vi "SimpleSetMotor.vi"(8 "error in (no error)":errorcluster, 10 "Output":dbl, 11 "MotorControlDevRef":T1={"DeviceStatus"={"status"=FALSE, "code"=0, "source"=""}, "Type"=enum."PWM", "PWM"={"Digital Module"=enum."Digital Module 1", "PWM Channel"=enum."Invalid", "DeadBand"={"Name"="", "maxPositivePwm"=0, "minPositivePwm"=0, "centerPwm"=0, "maxNegativePwm"=0, "minNegativePwm"=0, "angularRange"=0}}, "CAN"={"Device Number"=0, "Control Mode"=enum."Percent VBus", "Semaphore"=refnum, "Max Vout"=12.0}, "Invert"=FALSE, "TransformRef"=refnum, "InvTransformRef"=refnum}) -> (0 "error out":errorcluster, 3 "MotorControlDevRef":T1={"DeviceStatus"={"status"=FALSE, "code"=0, "source"=""}, "Type"=enum."PWM", "PWM"={"Digital Module"=enum."Digital Module 1", "PWM Channel"=enum."Invalid", "DeadBand"={"Name"="", "maxPositivePwm"=0, "minPositivePwm"=0, "centerPwm"=0, "maxNegativePwm"=0, "minNegativePwm"=0, "angularRange"=0}}, "CAN"={"Device Number"=0, "Control Mode"=enum."Percent VBus", "Semaphore"=refnum, "Max Vout"=12.0}, "Invert"=FALSE, "TransformRef"=refnum, "InvTransformRef"=refnum})   [LabVIEW 2011]
doc: "Specifies the output value or set-point for the motor controller.\n\nIf you use a Jaguar or Victor motor controller connected to PWM, the scaled value can range from -1.0 to 1.0.\n\nIf you use a CAN Jaguar, the scale and the units depend on the mode the Jaguar is in. In <B>Percent VBus</B> mode, the range is the same as the PWM interface. In <B>Voltage</B>, <B>Current</B>, <B>Speed</B>, and <B>Position</B> modes, the <B>Output</B> is specified in engineering units (Volts, Amps, Rotations/Minute, and Rotations respectively).\n\nThe output value can be modified by custom scaling if you specify the <B>TransformRef</B> VI reference in the Open VI. Use this transform if you need to apply a non-linear transformation to the motor control signal to compensate for the characteristics of the motor.\n\nThis software is licensed. Open the labview\\readme\\WPI Robotics Library Open Source License.txt file for more information."
uses:
  <vilib>/Rock Robotics/WPI/MotorControl/WPI_MotorControlDeviceRef.ctl
  <vilib>/Rock Robotics/SystemInterfaces/Typedef/FPGA_TypedefDigitalModule.ctl
  <vilib>/Rock Robotics/SystemInterfaces/DIO/FPGA_DIOPWMChannel.ctl
  <vilib>/Rock Robotics/WPI/PWM/WPI_PWMDeadband.ctl
  <vilib>/Rock Robotics/WPI/CAN/Jaguar/SubVIs/WPI_CANJaguar_ControlMode.ctl
  <vilib>/Rock Robotics/WPI/PWM/WPI_PWMTransform_ConPane.ctl
  <vilib>/Rock Robotics/SystemInterfaces/DIO/FPGA_DIODevRef.ctl
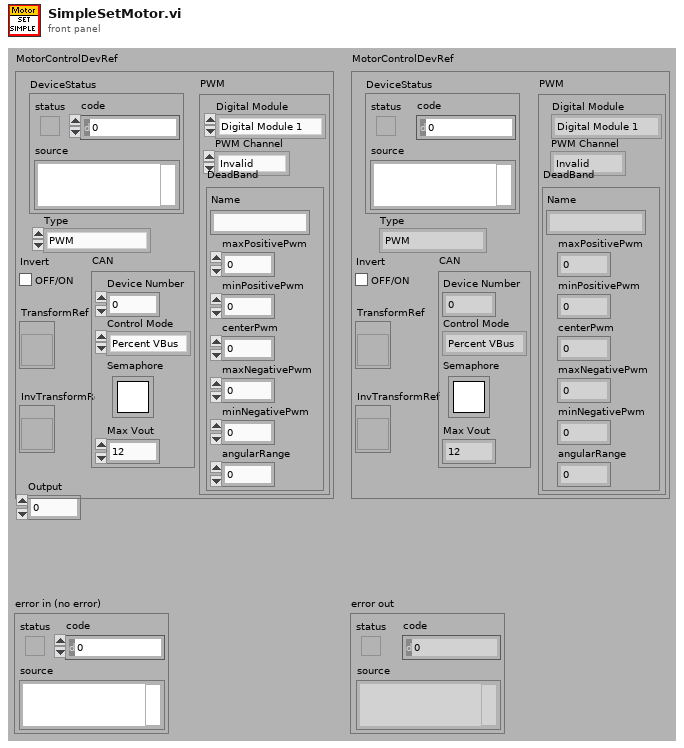
[diagram p1: front panel]
types:
  T1 = typedef "WPI_MotorControlDeviceRef.ctl" = cluster{"DeviceStatus":errorcluster, "Type":enum16{"PWM", "CAN"}, "PWM":cluster{"Digital Module":T2, "PWM Channel":T3, "DeadBand":T4}, "CAN":cluster{"Device Number":u8, "Control Mode":T5, "Semaphore":T6, "Max Vout":dbl}, "Invert":bool, "TransformRef":T7, "InvTransformRef":T7}
  T2 = typedef "FPGA_TypedefDigitalModule.ctl" = enum16{"Digital Module 1", "Digital Module 2"}
  T3 = typedef "FPGA_DIOPWMChannel.ctl" = enum8{"PWM 1", "PWM 2", "PWM 3", "PWM 4", "PWM 5", "PWM 6", "PWM 7", "PWM 8", "PWM 9", "PWM 10", "Invalid"}
  T4 = typedef "WPI_PWMDeadband.ctl" = cluster{"Name":string, "maxPositivePwm":i32, "minPositivePwm":i32, "centerPwm":i32, "maxNegativePwm":i32, "minNegativePwm":i32, "angularRange":u16}
  T5 = typedef "WPI_CANJaguar_ControlMode.ctl" = enum8{"Percent VBus", "Current", "Speed", "Position", "Voltage"}
  T6 = typedef "Semaphore RefNum" = refnum<k1>
  T7 = typedef "WPI_PWMTransform_ConPane.ctl" = refnum<vi>
  T8 = typedef "FPGA_DIODevRef.ctl" = cluster{"DevStatus":errorcluster, "Module":T2}
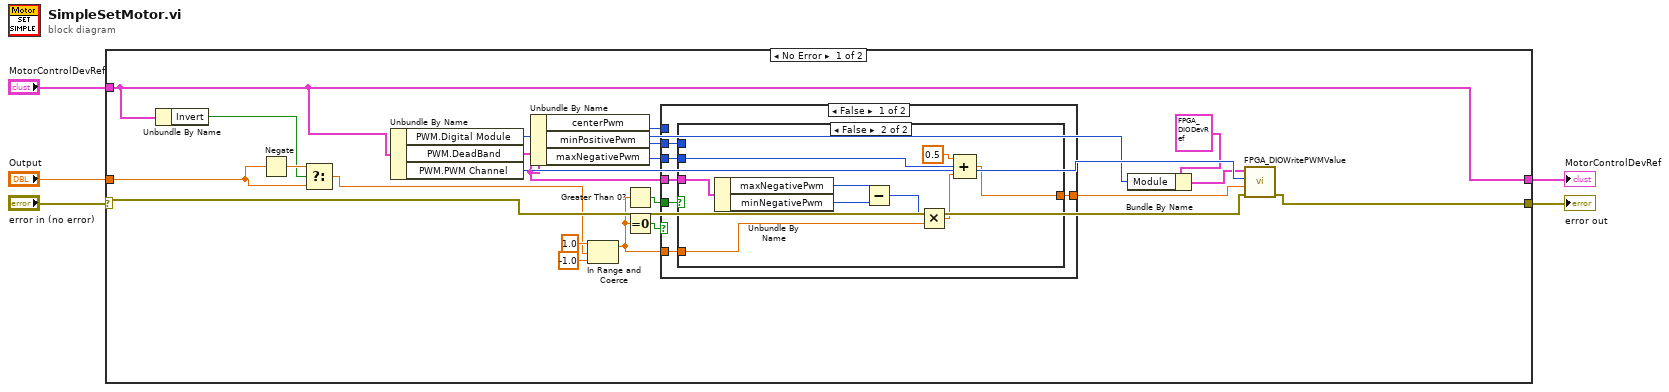
[diagram p0: block diagram]
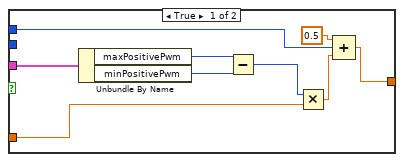
[diagram p2: hidden frame]
diagram:
  n1 = case shown="No Error" "error in (no error)" {
    selector: "error in (no error)" -> [w22 w53]
    tunnel: "MotorControlDevRef" -> [w24 w52]
    tunnel: [w24 w52] -> w1
    tunnel: "Output" -> [w21 _]
    tunnel: [w23 w53] -> w2
    frame No Error {
      n2 = Unbundle By Name(w24) -> ("Invert"=w25:bool)
      n3 = Negate(x=w21) -> (-x=w26:dbl)
      n4 = Select(t=w26, s=w25, f=w21) -> (s? t:f=w7:dbl)
      n5 = Unbundle By Name(w24) -> ("PWM.Digital Module"=w17:T2, "PWM.DeadBand"=w6:T4, "PWM.PWM Channel"=w20:T3)
      n6 = Unbundle By Name(w6) -> ("centerPwm"=w14:i32, "minPositivePwm"=w15:i32, "maxNegativePwm"=w16:i32)
      n7 = In Range and Coerce(upper limit=1.0, x=w7, lower limit=-1.0) -> (coerced(x)=w9:dbl)  [unwired: 1 out]
      n8 = Greater Than 0?(x=w9) -> (x > 0?=w10:bool)
      n9 = Equal To 0?(x=w9) -> (x = 0?=w11:bool)
      n10 = case shown="False" w11 {
        tunnel: w10 -> [w32 _]
        tunnel: w9 -> [w31 _]
        tunnel: w15 -> [w30 _]
        tunnel: w16 -> [w29 _]
        tunnel: [w28 w51] -> w8
        tunnel: w14 -> [_ w51]
        tunnel: w6 -> [w27 _]
        frame False {
          n11 = case shown="False" w32 {
            tunnel: w31 -> [w41 w50]
            tunnel: w30 -> [w39 _]
            tunnel: w29 -> [_ w46]
            tunnel: [w37 w47] -> w28
            tunnel: w27 -> [w33 w42]
            frame True {
              n12 = Unbundle By Name(w33) -> ("maxPositivePwm"=w35:i32, "minPositivePwm"=w36:i32)
              n13 = Subtract(x=w35, y=w36) -> (x-y=w34:i32)
              n14 = Multiply(x=w34, y=w41) -> (x*y=w40:dbl)
              n15 = Compound Arithmetic op=ADD(0.5 ("value"), w39, w40) -> (w37:dbl)
            }
            frame False {
              n16 = Unbundle By Name(w42) -> ("maxNegativePwm"=w44:i32, "minNegativePwm"=w45:i32)
              n17 = Subtract(x=w44, y=w45) -> (x-y=w43:i32)
              n18 = Multiply(x=w43, y=w50) -> (x*y=w49:dbl)
              n19 = Compound Arithmetic op=ADD(0.5 ("value"), w46, w49) -> (w47:dbl)
            }
          }
        }
        frame True {
        }
      }
      n20 = Bundle By Name(cluster=T8 {"DevStatus"={"status"=FALSE, "code"=0, "source"=""}, "Module"=enum."Digital Module 1"} ("DIODeviceRef In"), "Module"=w17) -> (w18:T8)
      n21 = call <vilib>:"FPGA_DIOWritePWMValue.vi"("error in (no error)"=w22, "PWMValue"=w8, "PWMChannel"=w20, "DIODeviceRef In"=w18) -> ("error out"=w23:errorcluster)  [unwired: 7 out]
    }
    frame Error {
    }
  }
  "MotorControlDevRef" <- w1
  "error out" <- w2
